vi "Add Malleable VI in Logic - Single Converter.vi"(0 "logic vi":refnum<vi>, 5 "sub vis ref":refnum<vi>[](array[refnum]), 11 "error in":errorcluster) -> (15 "error out":errorcluster)   [LabVIEW 2021, in "Converter.lvlib"]
uses:
  Converter.lvlib
  <vilib>/Utility/miscctls.llb/LVPointTypeDef.ctl
  <vilib>/ErrorRing/Error Ring.xnode
  Converter Reusables/Converter Reusables.lvlib
  Path Functions/Path Functions.lvlib
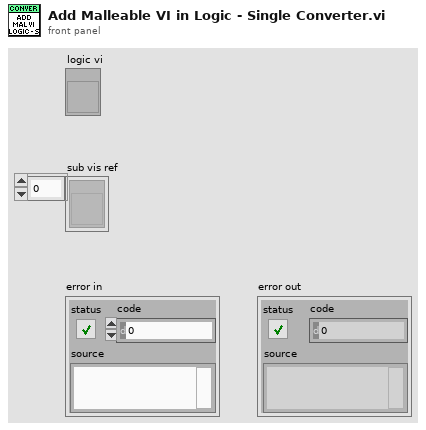
[diagram p1: front panel]
types:
  T1 = typedef "LVPointTypeDef.ctl" = cluster{"Horizontal":i16, "Vertical":i16}
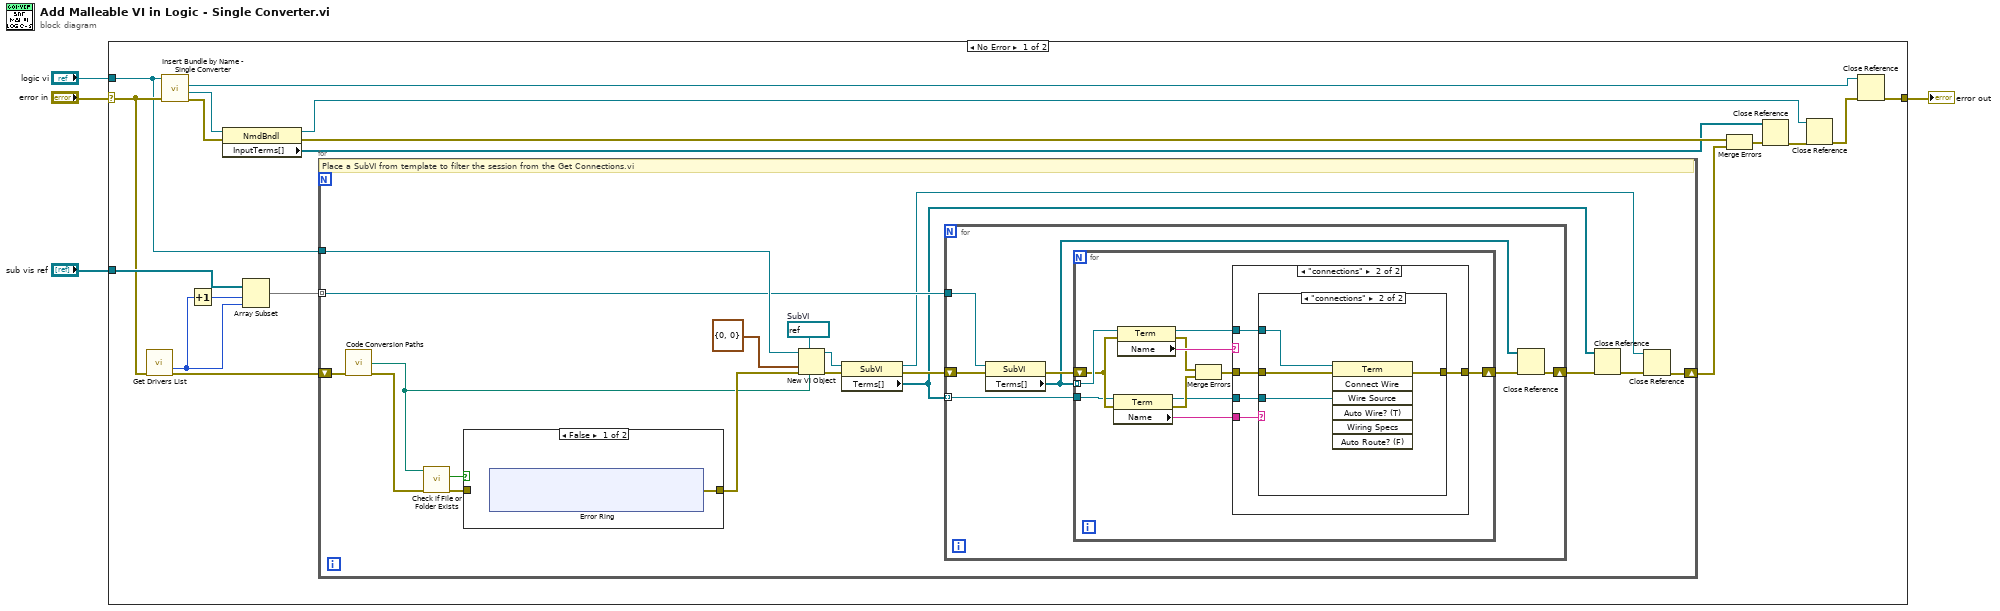
[diagram p0: block diagram]
diagram:
  n1 = case shown="No Error" "error in" {
    selector: "error in" -> [w12 w73]
    tunnel: [w22 w73] -> w4
    tunnel: "sub vis ref" -> [w13 _]
    tunnel: "logic vi" -> [w8 _]
    frame No Error {
      n2 = call "Get Drivers List.vi"("error in"=w12) -> ("removed duplicates size"=w6:i32, "error out"=w9:errorcluster)  [unwired: 9 in, 4 out]
      n3 = call "Insert Bundle by Name - Single Converter.vi"("error in"=w12, "vi in"=w8) -> ("error out"=w16:errorcluster, "named bundler"=w19:refnum<vi>, "wrapper refnum"=w21:refnum<vi>)  [unwired: 7 in]
      n4 = Increment(x=w6) -> (x+1=w5:i32)
      n5 = property on="Property Node" class="NmdBndl"(reference=w19, error in=w16) -> (reference out=w14:refnum<vi>, error out=w15:errorcluster, "InputTerms[]"=w11:refnum<vi>[])
      n6 = Array Subset(array=w13, index=w5, length=w6) -> (w10:refnum<vi>[])
      n7 = for {
        tunnel: w10 -> [w35] mode=indexing
        tunnel: w8 -> [w38]
        shift-right: [w30] -> w7
        shift-left: w9 -> [w40]
        w39 = refnum<vi> refnum  # SubVI
        # "Place a SubVI from template to filter the session from the Get Connections.vi"
        n8 = call "Code Conversion Paths.vi"("error in"=w40) -> ("get resource vi"=w23:path, "error out"=w25:errorcluster)  [unwired: 6 in, 7 out]
        n9 = call <vilib>:"Check if File or Folder Exists.vi"("error in (no error)"=w25, "path"=w23) -> ("error out"=w26:errorcluster, "file or folder exists?"=w27:bool)  [unwired: 7 in, 1 out]
        n10 = case shown="False" w27 {
          tunnel: w26 -> [_ w72]
          tunnel: [w70 w72] -> w24
          frame False {
            n11 = xnode ("Error Ring")() -> ("error out"=w70:errorcluster)
          }
          frame True {
          }
        }
        n12 = New VI Object(vi object class=w39, owner refnum=w38, position/next to=T1 {"Horizontal"=0, "Vertical"=0} ("location"), 6:w23, 8:w24) -> (object refnum=w31:refnum<vi>, 0:w37:errorcluster)  [unwired: 3 in]
        n13 = property on="Property Node" class="SubVI"(reference=w31, error in=w37) -> (reference out=w28:refnum<vi>, error out=w36:errorcluster, "Terms[]"=w33:refnum<vi>[])
        n14 = for {
          tunnel: w33 -> [w44] mode=indexing
          tunnel: w35 -> [w47]
          shift-right: [w41] -> w34
          shift-left: w36 -> [w46]
          n15 = property on="Property Node" class="SubVI"(reference=w47, error in=w46) -> (error out=w45:errorcluster, "Terms[]"=w42:refnum<vi>[])  [unwired: 1 out]
          n16 = for {
            tunnel: w42 -> [w58] mode=indexing
            tunnel: w44 -> [w56]
            shift-right: [w48] -> w43
            shift-left: w45 -> [w57]
            n17 = property on="Property Node" class="Term"(reference=w56, error in=w57) -> (reference out=w49:refnum<vi>, error out=w52:errorcluster, "Name"=w54:string)
            n18 = property on="Property Node" class="Term"(reference=w58, error in=w57) -> (reference out=w50:refnum<vi>, error out=w53:errorcluster, "Name"=w55:string)
            n19 = Merge Errors(w53, w52) -> (w51:errorcluster)
            n20 = case shown="\"connections\"" w55 {
              tunnel: w54 -> [_ w64]
              tunnel: w51 -> [w59 w62]
              tunnel: w50 -> [_ w63]
              tunnel: w49 -> [_ w61]
              tunnel: [w59 w60] -> w48
              frame Default {
              }
              frame "connections" {
                n21 = case shown="\"connections\"" w64 {
                  tunnel: w63 -> [_ w69]
                  tunnel: w62 -> [w65 w68]
                  tunnel: w61 -> [_ w67]
                  tunnel: [w65 w66] -> w60
                  frame Default {
                  }
                  frame "connections" {
                    n22 = invoke on="Invoke Node" class="Term" method="Connect Wire"(reference=w69, error in=w68, "Wire Source"=w67) -> (error out=w66:errorcluster)  [unwired: 4 in, 6 out]
                  }
                }
              }
            }
          }
          n23 = Close Reference(reference=w42, error in (no error)=w43) -> (error out=w41:errorcluster)
        }
        n24 = Close Reference(reference=w33, error in (no error)=w34) -> (error out=w32:errorcluster)
        n25 = Close Reference(reference=w28, error in (no error)=w32) -> (error out=w30:errorcluster)
      }
      n26 = Merge Errors(w15, w7) -> (w18:errorcluster)
      n27 = Close Reference(reference=w11, error in (no error)=w18) -> (error out=w17:errorcluster)
      n28 = Close Reference(reference=w14, error in (no error)=w17) -> (error out=w20:errorcluster)
      n29 = Close Reference(reference=w21, error in (no error)=w20) -> (error out=w22:errorcluster)
    }
    frame Error {
    }
  }
  "error out" <- w4
